vi "TestDeviceListReadOut.vi"() -> ()   [LabVIEW 2023]
uses:
  DeviceManager.lvlib
  Classes/CCD/CCD.lvclass
panel:
  out "unformated list of devices":string[](array[string])
  out "Array":string[](array[string])
  out "table of devices":string[][](array[string])
  out "array":string[](array[string])
  out "List of devices 2":string[](array[string])
  # "Connector Pane"
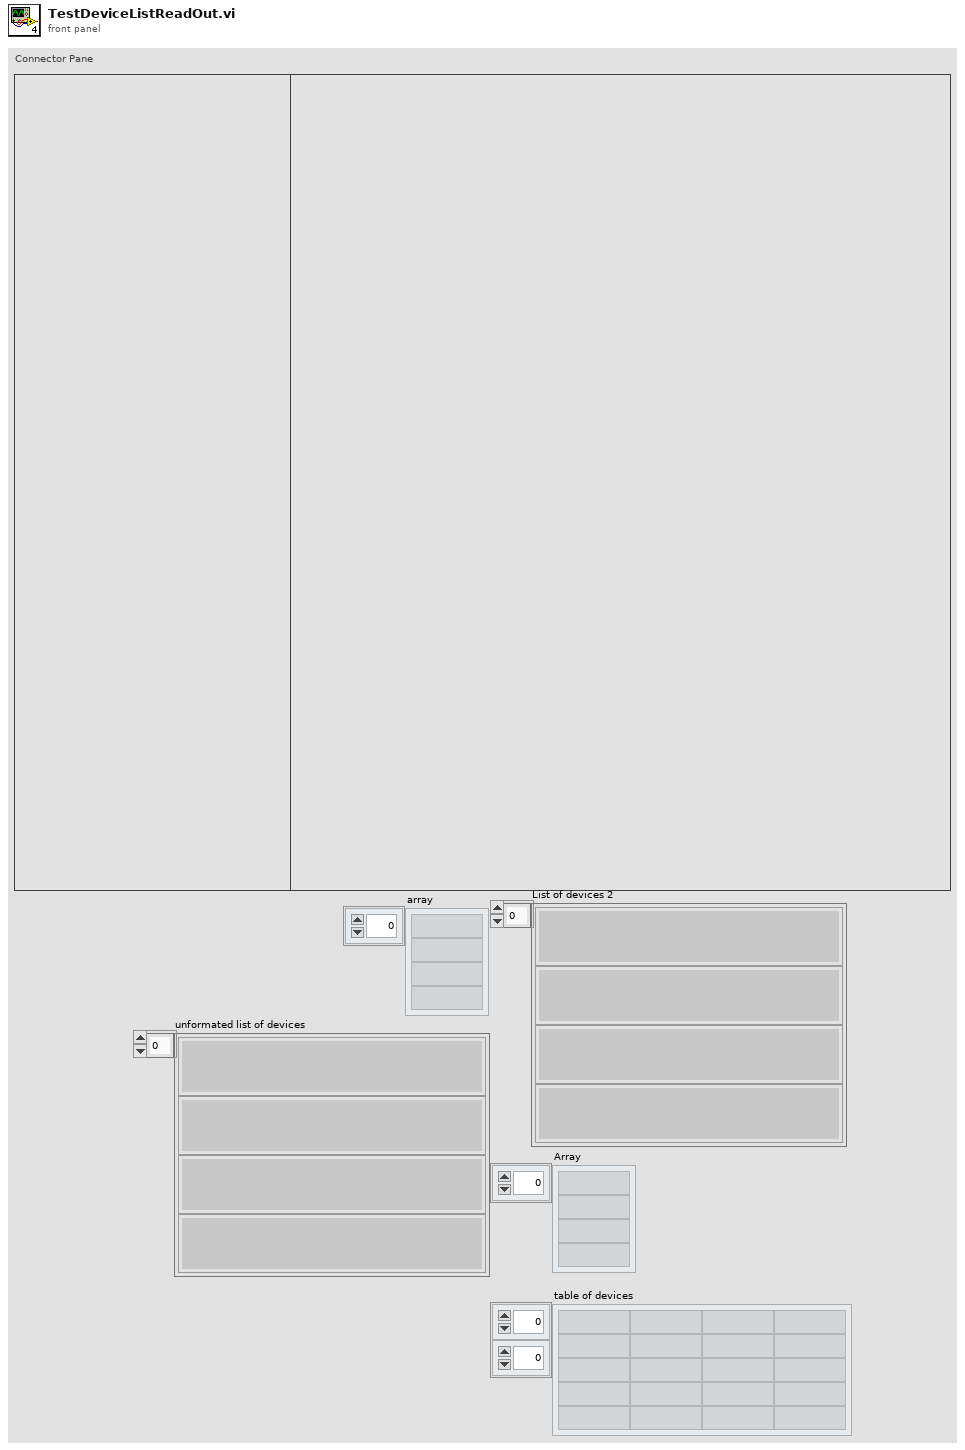
[diagram p1: front panel]
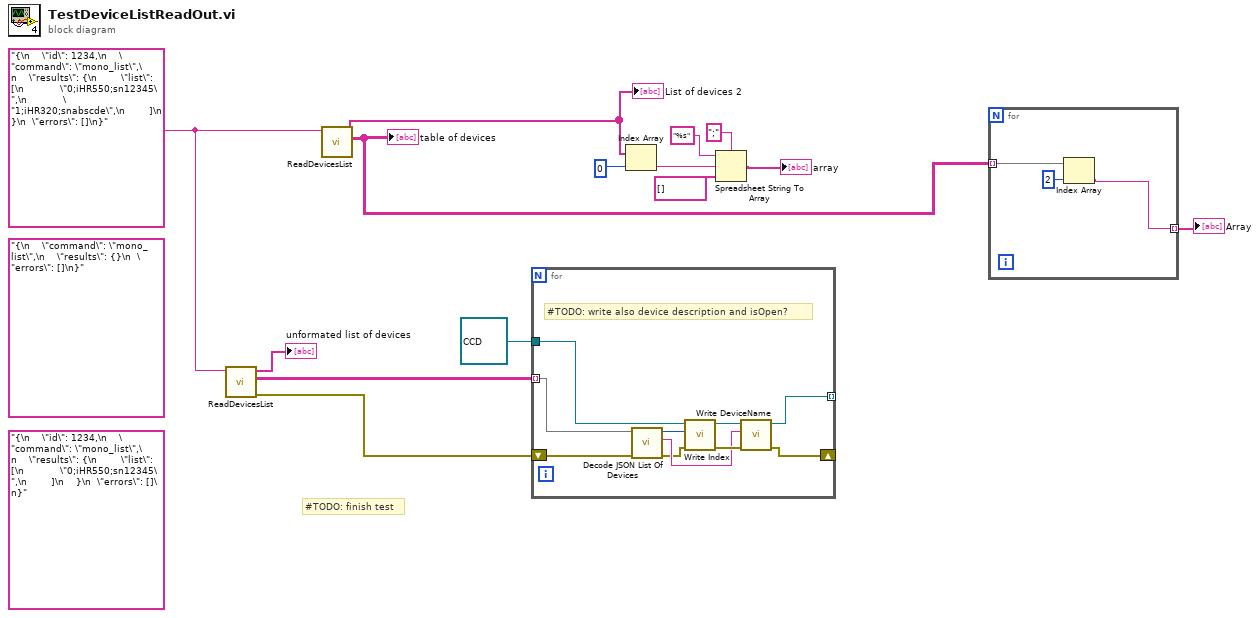
[diagram p0: block diagram]
diagram:
  (unwired) "{\n    \"id\": 1234,\n    \"command\": \"mono_list\",\n    \"results\": {\n        \"list\": [\n            \"0;iHR550;sn12345\",\n        ]\n    }\n  \"errors\": []\n}"
  (unwired) "{\n    \"command\": \"mono_list\",\n    \"results\": {}\n  \"errors\": []\n}"
  w1 = "{\n    \"id\": 1234,\n    \"command\": \"mono_list\",\n    \"results\": {\n        \"list\": [\n            \"0;iHR550;sn12345\",\n            \"1;iHR320;snabscde\",\n        ]\n    }\n  \"errors\": []\n}"
  # "#TODO: finish test"
  n1 = call "ReadDevicesList.vi"("JSON"=w1) -> ("error out"=w3:errorcluster, "table of devices"=w4:string[][], "unformated list of devices"=→"unformated list of devices":string[])  [unwired: 8 in]
  n2 = call "ReadDevicesList.vi"("JSON"=w1) -> ("table of devices"=w7:string[][], "unformated list of devices"=w8:string[])  [unwired: 8 in, 1 out]
  "List of devices 2" <- w8
  "table of devices" <- w7
  n3 = for {
    tunnel: w4 -> [w21] mode=indexing
    shift-right: [w17] -> _
    shift-left: w3 -> [w22]
    tunnel: [w16] -> _ mode=indexing
    tunnel: refnum<class "CCD.lvclass"> refnum ("CCD.lvclass") -> [w15]
    # "#TODO: write also device description and isOpen?"
    n4 = call "Decode JSON List Of Devices.vi"("error in"=w22, "table of devices"=w21) -> ("error out"=w18:errorcluster, "name of device"=w19:string, "device index"=w20:i32)  [unwired: 6 in, 1 out]
    n5 = call-dynamic "Write Index.vi"("error in (no error)"=w18, "Index"=w20, "CCD in"=w15) -> ("error out"=w23:errorcluster, "CCD out"=w24:refnum<class "CCD.lvclass">)  [unwired: 7 in]
    n6 = call-dynamic "Write DeviceName.vi"("error in (no error)"=w23, "DeviceName"=w19, "CCD in"=w24) -> ("error out"=w17:errorcluster, "CCD out"=w16:refnum<class "CCD.lvclass">)  [unwired: 7 in]
  }
  n7 = Index Array(array=w8, index=0) -> (element=w13:string)
  n8 = Spreadsheet String To Array(delimiter (Tab)=";", format string="%s", spreadsheet string=w13, array type (2D Dbl)=string[] []) -> (array=→"array":string[])
  n9 = for {
    tunnel: w7 -> [w27] mode=indexing
    tunnel: [w26] -> w6 mode=indexing
    n10 = Index Array(array=w27, index=2) -> (element=w26:string)
  }
  "Array" <- w6
